vi "ROSServiceRead.vi"(0 "error in":errorcluster, 1 "vi reference":refnum<vi>) -> (2 "error out":errorcluster, 3 "Reply":string, 4 "vi reference":refnum<vi>)   [LabVIEW 2010]
doc: "Attempts to wait for a response from a server call before returning an empty string. Implemented in ROS_Topic_Read."
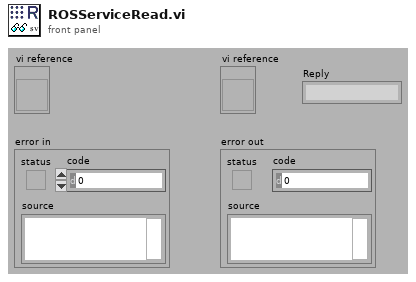
[diagram p1: front panel]
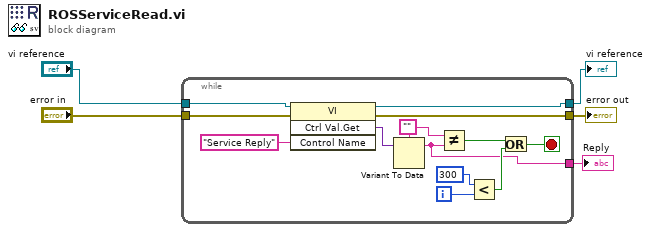
[diagram p0: block diagram]
diagram:
  n1 = while {
    tunnel: "vi reference" -> [w18]
    tunnel: [w17] -> w4
    tunnel: [w16] -> w5
    tunnel: "error in" -> [w15]
    tunnel: [w6] -> w3
    i -> [w12]
    stop <- w9 stop-if-true
    w8 = ""
    n2 = invoke class="VI" method="Ctrl Val.Get"(reference=w18, error in=w15, "Control Name"="Service Reply") -> (reference out=w17:refnum<vi>, error out=w16:errorcluster, "Get Control Value Variant"=w13:variant)  [unwired: 1 in, 1 out]
    n3 = Variant To Data(Variant=w13, type=w8) -> (data=w6:string)  [unwired: 1 in, 1 out]
    n4 = Not Equal?(x=w8, y=w6) -> (x != y?=w7:bool)
    n5 = Less?(x=300, y=w12) -> (x < y?=w10:bool)
    n6 = Or(x=w7, y=w10) -> (x .or. y?=w9:bool)
  }
  "error out" <- w5
  "vi reference" <- w4
  "Reply" <- w3
